vi "Write to file API.vi"(8 "Error In":errorcluster, 10 "Waveform name":string, 11 "Waveform Data":dbl[][](array[numeric])) -> (0 "Error Out":errorcluster)   [LabVIEW 2017, in "DAQ.lvlib"]
uses:
  DAQ.lvlib
  Controls/Command Data [cluster].ctl
  Controls/Commands [enum].ctl
  Events/Events.lvlib
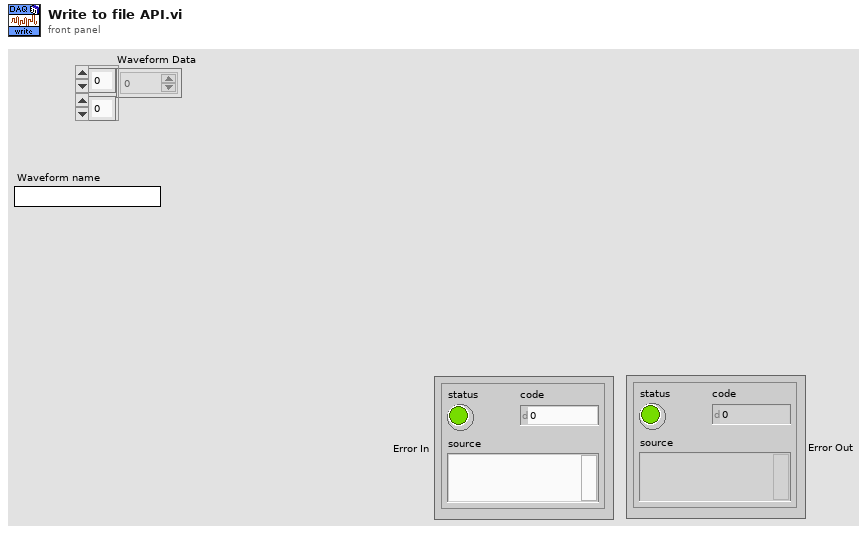
[diagram p1: front panel]
types:
  T1 = typedef "DAQ.lvlib/Command Data [cluster].ctl" = cluster{"Command":T2, "Data":variant}
  T2 = typedef "DAQ.lvlib/Commands [enum].ctl" = enum16{"Calculate parameters", "Start", "Stop", "Get test data", "Accumulate test data", "Average test data", "Calculate background voltage", "Send data", "Write data to file"}
  T3 = cluster{"Waveform Data":dbl[][], "Waveform name":string}
  T4 = typedef "Events.lvlib/Refs [cluster].ctl" = cluster{"Exit":refnum<user-event>, "Controller":refnum<user-event>, "System Error":refnum<user-event>, "UI":refnum<user-event>, "Example Module":refnum<user-event>, "Shutter":refnum<user-event>, "Monochromator":refnum<user-event>, "DAQ":refnum<user-event>, "Scope":refnum<user-event>, "Processing":refnum<user-event>, "File IO":refnum<user-event>, "Colour wheel":refnum<user-event>}
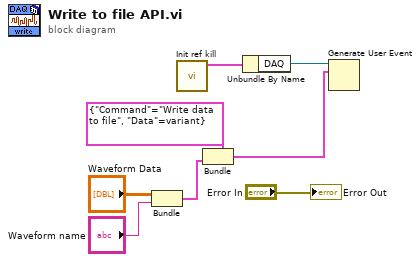
[diagram p0: block diagram]
diagram:
  n1 = Bundle("Waveform Data"="Waveform Data", "Waveform name"="Waveform name") -> (w3:T3)  [unwired: 1 in]
  n2 = call "Init ref kill.vi"() -> ("Messages"=w8:T4)  [unwired: 10 in, 1 out]
  n3 = Bundle(cluster=T1 {"Command"=enum."Write data to file", "Data"=variant} ("event data"), "Data"=w3) -> (w4:T1)  [unwired: 1 in]
  n4 = Unbundle By Name(w8) -> ("DAQ"=w7:refnum<user-event>)
  n5 = Generate User Event(user event=w7, event data cluster=w4) -> ()  [unwired: 2 in, 2 out]
  "Error Out" <- "Error In"
